vi "CRYPIC PreGetVIName.vi"(9 "sVIName":string) -> (0 "sData_Out":string, 1 "sVIName_Out":string)   [LabVIEW 2013]
panel:
  # "Split Parameter Name."
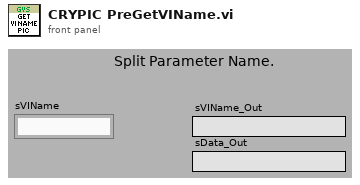
[diagram p1: front panel]
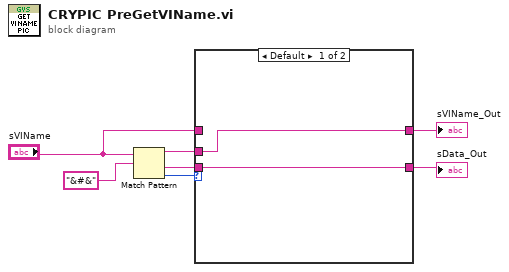
[diagram p0: block diagram]
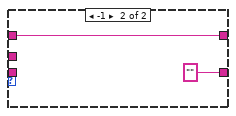
[diagram p2: hidden frame]
diagram:
  n1 = Match Pattern(string="sVIName", regular expression="&#&") -> (before substring=w5:string, after substring=w4:string, offset past match=w6:i32)  [unwired: 1 in, 1 out]
  n2 = case shown="Default" w6 {
    tunnel: "sVIName" -> [_ w11]
    tunnel: w5 -> [w9 _]
    tunnel: w4 -> [w8 _]
    tunnel: [w9 w11] -> w3
    tunnel: [w8 "" ("sVIName")] -> w2
    frame Default {
    }
    frame -1 {
    }
  }
  "sVIName_Out" <- w3
  "sData_Out" <- w2
